vi "Handle Error.vi"(7 "Stop on Unhandled Error (T)":bool=TRUE, 8 "error in":errorcluster, 11 "SMO.ErrorInjection":refnum<class "SMO.ErrorInjection.lvclass">) -> (0 "handling error":errorcluster, 2 "Unhandled error":errorcluster, 3 "SMO.ErrorInjection out":refnum<class "SMO.ErrorInjection.lvclass">)   [LabVIEW 2013, in "SMO.ErrorInjection.lvclass"]
doc: "JKI State Machine Objects (SMO) 1.0.0.11\nJKI - JKI\nCopyright (c) 2016, JKI"
uses:
  SMO.ErrorInjection.lvclass
  src/SMO/SMO.lvclass
panel:
  # "For instructions on how to use the JKI State Machine Objects, examples and video tutorials, visit:\nhttp://jki.net/state-machine-objects/\n\nJKI State Machine Objects™\nhttp://jki.net/state-machine-objects/\nCopyright (C) 2005-2015, JKI <info@jki.net>\nALL RIGHTS RESERVED"
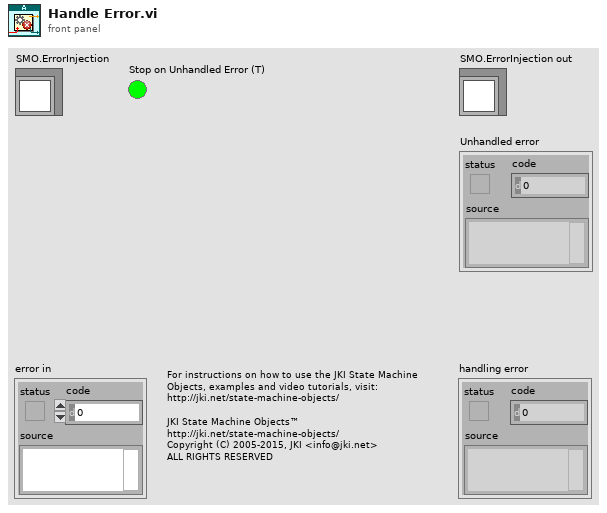
[diagram p1: front panel]
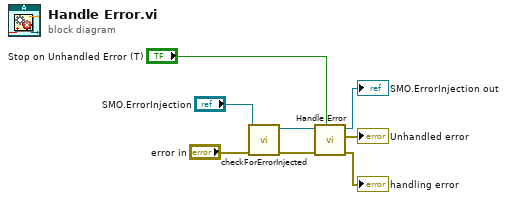
[diagram p0: block diagram]
diagram:
  n1 = call "checkForErrorInjected.vi"("error in (no error)"="error in", "SMO.ErrorInjection in"="SMO.ErrorInjection") -> ("error out"=w1:errorcluster, "SMO.ErrorInjection dup"=w3:refnum<class "SMO.ErrorInjection.lvclass">)  [unwired: 8 in]
  n2 = call-parent "Handle Error.vi"("Stop on Unhandled Error (T)"="Stop on Unhandled Error (T)", "error in"=w1, "SMO"=w3) -> ("handling error"=→"handling error":errorcluster, "Unhandled error"=→"Unhandled error":errorcluster, "SMO out"=→"SMO.ErrorInjection out":refnum<class "SMO.ErrorInjection.lvclass">)  [unwired: 6 in]
